vi "Get Sample Clock Rate.vi"(0 "device session in":refnum<class "Device Session.lvclass">, 11 "error in":errorcluster) -> (4 "device session out":refnum<class "Device Session.lvclass">, 6 "sample clock rate (Hz)":dbl, 15 "error out":errorcluster)   [LabVIEW 2015, in "Device Session.lvclass"]
doc: "Returns the sample rate of the configured clock.\n\n[paramName]\ndevice session in\n\n[paramDescription]\nis a reference to the session containing sessions to all instrument design libraries used in this sample project. This parameter is obtained from the <B>Open Session</B> VI.\n\n[paramName]\nerror in\n\n[paramDescription]\ndescribes error conditions that occur before this node runs. This input provides standard <b>error in</b> functionality.\n\n[outputParameters]\n\n[paramName]\ndevice session out\n\n[paramDescription]\npasses a reference to the session to the next VI.\n\n[paramName]\nsample clock rate (Hz)\n[paramDescription]\nis the sample rate of the configured clock.\n\n[paramName]\nerror out\n\n[paramDescription]\ncontains error information. This output provides standard <b>error out</b> functionality."
uses:
  Device Session.lvclass
  Device Session.lvclass/Device Session.ctl
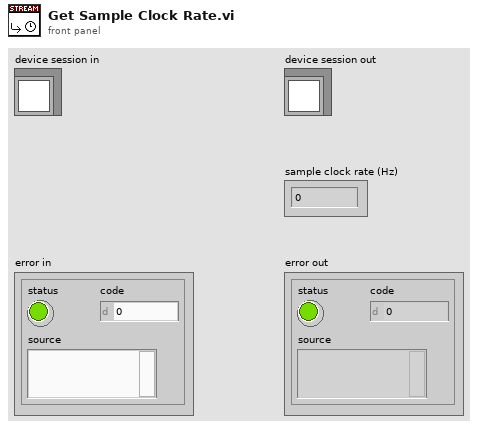
[diagram p1: front panel]
types:
  T1 = typedef "Device Session.lvclass/Device Session Object.ctl" = cluster{"ni5171R FPGA Reference":T2, "niHSAI config":refnum<class "niHSAI Config v1 Host.lvclass">, "configured scaling coefficients":cluster{"gain":dbl, "offset":dbl}[], "number of channels to stream":u8, "selected acq channels":bool[], "number of channels":u32, "actual channel configuration":T3[], "configured channels":bool[], "sample clock rate (Hz)":dbl}
  T2 = typedef "Device Session.lvclass/FPGA Refnum.ctl" = refnum<k20>
  T3 = typedef "niHSAI Types v1 Host.lvlib/Channel Configuration.ctl" = cluster{"channel":u32, "coupling":T4, "impedance":T5, "bandwidth":T6, "vertical range":dbl, "vertical offset":dbl}
  T4 = typedef "niHSAI Types v1 Host.lvlib/Coupling.ctl" = enum8{"Default", "DC", "AC"}
  T5 = typedef "niHSAI Types v1 Host.lvlib/Impedance.ctl" = enum8{"Default", "1 mega ohm", "50 ohm"}
  T6 = typedef "niHSAI Types v1 Host.lvlib/Bandwidth.ctl" = enum8{"Default", "Full Bandwidth", "Anti-alias Filter"}
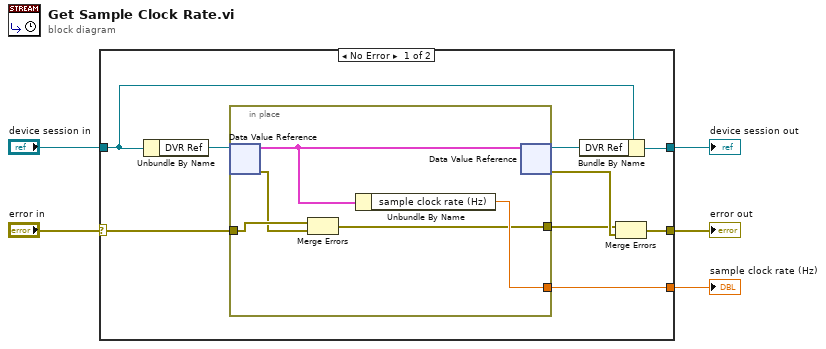
[diagram p0: block diagram]
diagram:
  n1 = case shown="No Error" "error in" {
    selector: "error in" -> [w14 w21]
    tunnel: [w9 w21] -> w2
    tunnel: "device session in" -> [w11 w20]
    tunnel: [w10 w20] -> w3
    tunnel: [w7 _] -> w1
    frame No Error {
      n2 = Unbundle By Name(w11) -> ("DVR Ref"=w13:refnum<data-value>)
      n3 = in-place {
        in-place-border: w14 -> [w19]
        in-place-border: [w16] -> w7
        in-place-border: [w15] -> w6
        n4 = in-place-dvr #1(w13) -> (w17:T1, w18:errorcluster)
        n5 = Merge Errors(w19, w18) -> (w15:errorcluster)
        n6 = Unbundle By Name(w17) -> ("sample clock rate (Hz)"=w16:dbl)
        n7 = in-place-dvr #1(w17) -> (w12:refnum<data-value>, w8:errorcluster)
      }
      n8 = Bundle By Name(cluster=w11, "DVR Ref"=w12) -> (w10:refnum<class "Device Session.lvclass">)
      n9 = Merge Errors(w6, w8) -> (w9:errorcluster)
    }
    frame Error {
    }
  }
  "error out" <- w2
  "device session out" <- w3
  "sample clock rate (Hz)" <- w1
